vi "Shooter RPM.vi"() -> (3 "RPM Output":dbl)   [LabVIEW 2011]
panel:
  out "RPM":cluster{dbl, dbl, dbl[]}(graph)
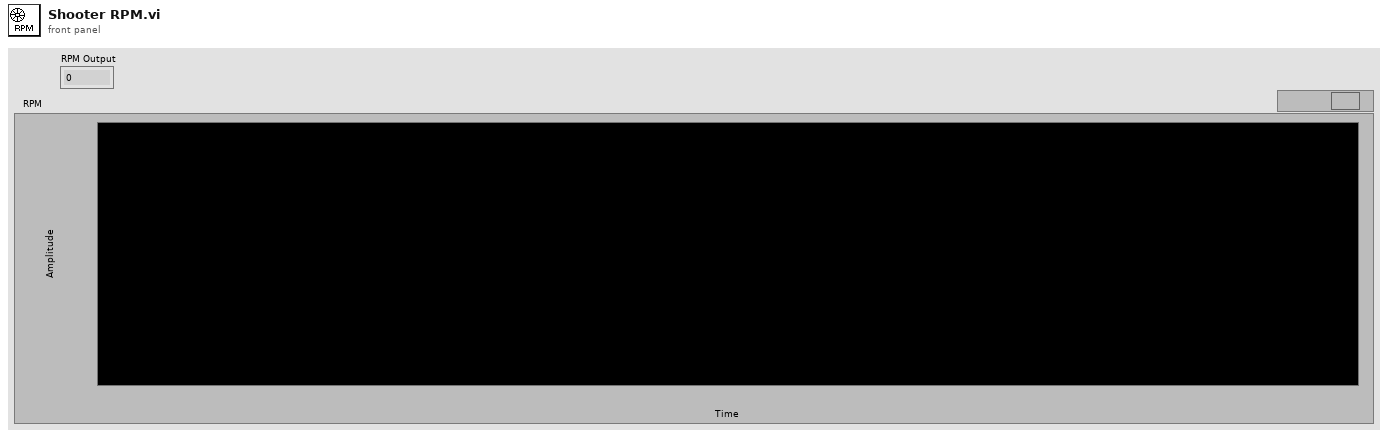
[diagram p1: front panel]
types:
  T1 = typedef "WPI_EncoderDevRef.ctl" = cluster{"DevStatus":errorcluster, "EncoderIndex":T2, "CounterIndex":T3, "DistancePerCount":dbl, "Decoding Type":T4}
  T2 = typedef "FPGA_EncoderIdx.ctl" = enum8{"Enc 0", "Enc 1", "Enc 2", "Enc 3", "Invalid"}
  T3 = typedef "FPGA_CounterCtrSystemIndex.ctl" = enum8{"Ctr 0", "Ctr 1", "Ctr 2", "Ctr 3", "Ctr 4", "Ctr 5", "Ctr 6", "Ctr 7", "Invalid"}
  T4 = typedef "WPI_EncoderType.ctl" = enum16{"1x", "2x", "4x"}
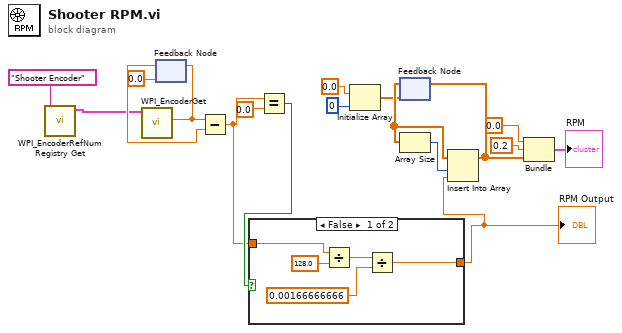
[diagram p0: block diagram]
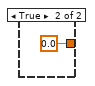
[diagram p2: hidden frame]
diagram:
  n1 = call <vilib>:"WPI_EncoderRefNum Registry Get.vi"("refnum name"="Shooter Encoder") -> ("EncoderDevRef"=w1:T1)  [unwired: 9 in, 1 out]
  n2 = call <vilib>:"WPI_EncoderGet.vi"("EncoderDevRef"=w1) -> ("Distance"=w7:dbl)  [unwired: 5 in, 5 out]
  n3 = feedback #1(0.0) -> (w10:dbl)
  n4 = feedback-in #1(w7) -> ()
  n5 = Subtract(x=w7, y=w10) -> (x-y=w4:dbl)
  n6 = Equal?(x=w4, y=0.0) -> (x = y?=w5:bool)
  n7 = case shown="False" w5 {
    tunnel: [w20 0.0] -> w3
    tunnel: w4 -> [w19 _]
    frame False {
      n8 = Divide(x=w19, y=128.0) -> (x/y=w22:dbl)
      n9 = Divide(x=w22, y=0.00166666666) -> (x/y=w20:dbl)
    }
    frame True {
    }
  }
  "RPM Output" <- w3
  n10 = Initialize Array(0.0 ("element"), 0 ("dimension size")) -> (w13:dbl[])
  n11 = feedback #2(w13) -> (w14:dbl[])
  n12 = Array Size(array=w14) -> (size(s)=w15:i32)
  n13 = Insert Into Array(array=w14, index=w15, new element=w3) -> (w18:dbl[])
  n14 = feedback-in #2(w18) -> ()
  n15 = Bundle(0.0, 0.2, w18) -> (→"RPM":cluster{dbl, dbl, dbl[]})  [unwired: 1 in]
